vi "Is an Actor-Interface.vi"(10 "Class in":refnum<vi>) -> (0 "AF Library FQN":string, 1 "Is Actor/Interface?":bool, 2 "Class out":refnum<vi>, 3 "Message Recipient Type":T1)   [LabVIEW 2023, in "Message Maker.lvclass"]
uses:
  Message Maker.lvclass
  Message Recipient Type.ctl
  Message Maker.lvclass/Message Maker.ctl
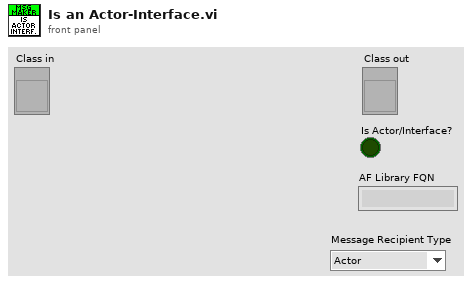
[diagram p1: front panel]
types:
  T1 = typedef "Message Maker.lvclass/Message Recipient Type.ctl" = enum16{"Actor", "Interface"}
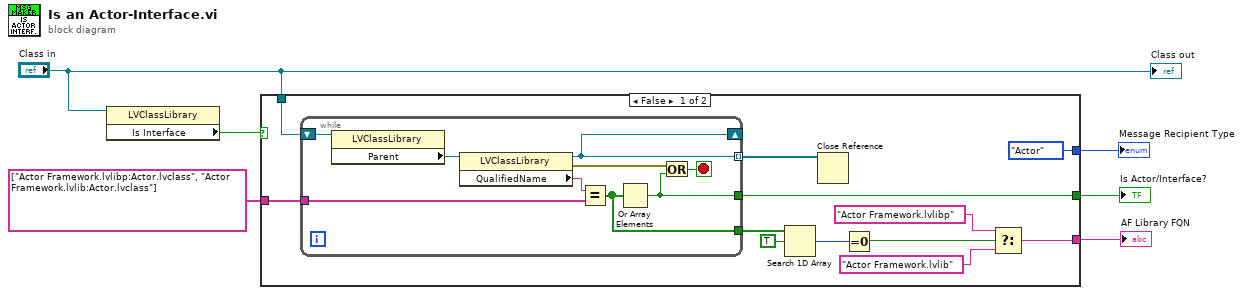
[diagram p0: block diagram]
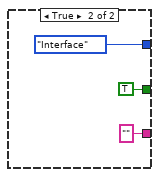
[diagram p2: hidden frame]
diagram:
  n1 = property class="LVClassLibrary"(reference="Class in") -> ("Is Interface"=w3:bool)  [unwired: 1 in, 2 out]
  n2 = case shown="False" w3 {
    tunnel: string[] ["Actor Framework.lvlibp:Actor.lvclass", "Actor Framework.lvlib:Actor.lvclass"] -> [w18 _]
    tunnel: [w10 "" ("Actor Class")] -> w5
    tunnel: "Class in" -> [w9 _]
    tunnel: [w8 TRUE] -> w2
    tunnel: [Message_Recipient_Type."Actor" ("Message Recipient Type") Message_Recipient_Type."Interface" ("Message Recipient Type")] -> w1
    frame False {
      n3 = while {
        shift-right: [w25] -> _
        shift-left: w9 -> [w27]
        tunnel: [w25] -> w17 mode=indexing
        tunnel: w18 -> [w23]
        tunnel: [w20] -> w8
        tunnel: [w19] -> w16
        stop <- w21 stop-if-true
        n4 = property class="LVClassLibrary"(reference=w27) -> ("Parent"=w26:refnum<vi>)  [unwired: 1 in, 2 out]
        n5 = property class="LVClassLibrary"(reference=w26) -> (reference out=w25:refnum<vi>, error out=w22:errorcluster, "QualifiedName"=w24:string)  [unwired: 1 in]
        n6 = Equal?(x=w24, y=w23) -> (x = y?=w19:bool[])
        n7 = Or Array Elements(Boolean array=w19) -> (logical OR=w20:bool)
        n8 = Or(x=w22, y=w20) -> (x .or. y?=w21:bool)
      }
      n9 = Search 1D Array(1D array=w16, element=TRUE) -> (index of element=w14:i32)  [unwired: 1 in]
      n10 = Close Reference(reference=w17) -> ()  [unwired: 1 in, 1 out]
      n11 = Equal To 0?(x=w14) -> (x = 0?=w13:bool)
      n12 = Select(t="Actor Framework.lvlibp" ("Actor Class"), s=w13, f="Actor Framework.lvlib" ("Actor Class")) -> (s? t:f=w10:string)
    }
    frame True {
    }
  }
  "AF Library FQN" <- w5
  "Is Actor/Interface?" <- w2
  "Message Recipient Type" <- w1
  "Class out" <- "Class in"
